vi "Get Variant Data From File.vi"(8 "error in (no error)":errorcluster, 10 "Variant Name":string, 11 "File refnum in":T1) -> (0 "error out":errorcluster, 2 "Variant Data Cluster":T2, 3 "File refnum out":T1)   [LabVIEW 2015]
uses:
  <vilib>/Utility/config.llb/Config Data RefNum.ctl
  Type defs/Variant Data Cluster.ctl
  <vilib>/Utility/config.llb/Read Key (String).vi
  <vilib>/Utility/config.llb/NI_LVConfig.lvlib
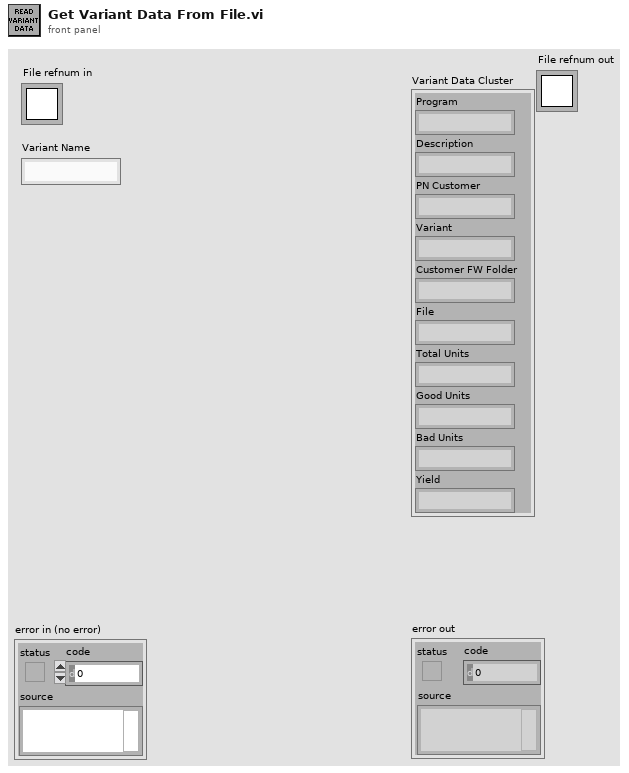
[diagram p1: front panel]
types:
  T1 = typedef "NI_LVConfig.lvlib/Config Data RefNum.ctl" = refnum<k1>
  T2 = typedef "Variant Data Cluster.ctl" = cluster{"Program":string, "Description":string, "PN Customer":string, "Variant":string, "Customer FW Folder":string, "File":string, "Total Units":string, "Good Units":string, "Bad Units":string, "Yield":string}
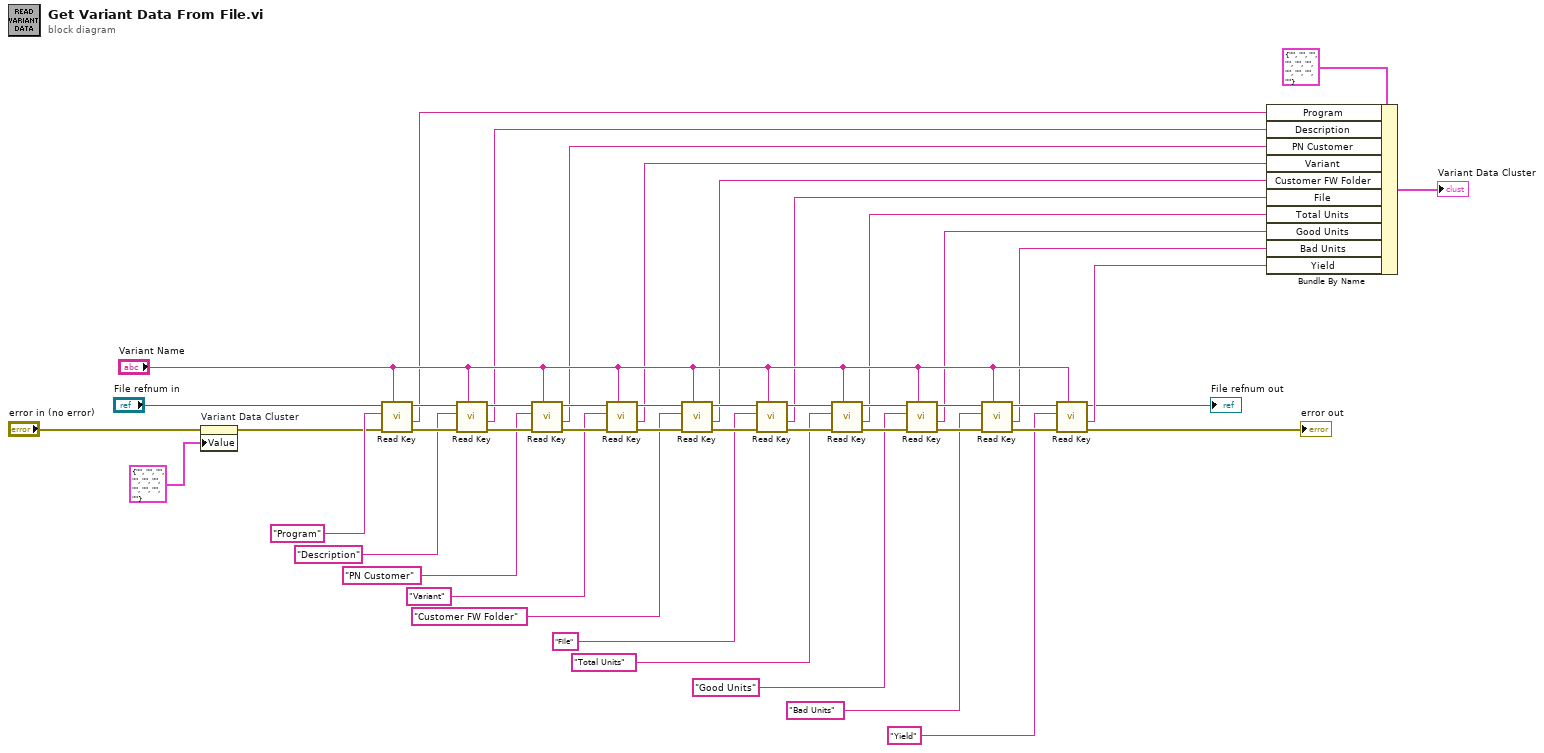
[diagram p0: block diagram]
diagram:
  n1 = property on="Variant Data Cluster" class="Clust (strict)"(error in="error in (no error)", "Value"=T2 {"Program"="", "Description"="", "PN Customer"="", "Variant"="", "Customer FW Folder"="", "File"="", "Total Units"="", "Good Units"="", "Bad Units"="", "Yield"=""} ("Variant Data Cluster")) -> (error out=w2:errorcluster)  [unwired: 1 in, 1 out]
  n2 = call-poly <vilib>:"Read Key.vi"("section"="Variant Name", "error in (no error)"=w2, "key"="Program", "refnum"="File refnum in") -> ("error out"=w43:errorcluster, "value"=w16:string, "refnum out"=w44:T1)  [unwired: 4 in, 1 out]
  n3 = call-poly <vilib>:"Read Key.vi"("section"="Variant Name", "error in (no error)"=w43, "key"="Description", "refnum"=w44) -> ("error out"=w42:errorcluster, "value"=w15:string, "refnum out"=w34:T1)  [unwired: 4 in, 1 out]
  n4 = call-poly <vilib>:"Read Key.vi"("section"="Variant Name", "error in (no error)"=w42, "key"="PN Customer", "refnum"=w34) -> ("error out"=w41:errorcluster, "value"=w14:string, "refnum out"=w33:T1)  [unwired: 4 in, 1 out]
  n5 = call-poly <vilib>:"Read Key.vi"("section"="Variant Name", "error in (no error)"=w41, "key"="Variant", "refnum"=w33) -> ("error out"=w40:errorcluster, "value"=w13:string, "refnum out"=w32:T1)  [unwired: 4 in, 1 out]
  n6 = call-poly <vilib>:"Read Key.vi"("section"="Variant Name", "error in (no error)"=w40, "key"="Customer FW Folder", "refnum"=w32) -> ("error out"=w39:errorcluster, "value"=w12:string, "refnum out"=w31:T1)  [unwired: 4 in, 1 out]
  n7 = call-poly <vilib>:"Read Key.vi"("section"="Variant Name", "error in (no error)"=w39, "key"="File", "refnum"=w31) -> ("error out"=w38:errorcluster, "value"=w11:string, "refnum out"=w30:T1)  [unwired: 4 in, 1 out]
  n8 = call-poly <vilib>:"Read Key.vi"("section"="Variant Name", "error in (no error)"=w38, "key"="Total Units", "refnum"=w30) -> ("error out"=w37:errorcluster, "value"=w10:string, "refnum out"=w29:T1)  [unwired: 4 in, 1 out]
  n9 = call-poly <vilib>:"Read Key.vi"("section"="Variant Name", "error in (no error)"=w37, "key"="Good Units", "refnum"=w29) -> ("error out"=w36:errorcluster, "value"=w9:string, "refnum out"=w28:T1)  [unwired: 4 in, 1 out]
  n10 = call-poly <vilib>:"Read Key.vi"("section"="Variant Name", "error in (no error)"=w36, "key"="Bad Units", "refnum"=w28) -> ("error out"=w35:errorcluster, "value"=w8:string, "refnum out"=w27:T1)  [unwired: 4 in, 1 out]
  n11 = call-poly <vilib>:"Read Key.vi"("section"="Variant Name", "error in (no error)"=w35, "key"="Yield", "refnum"=w27) -> ("error out"=→"error out":errorcluster, "value"=w7:string, "refnum out"=→"File refnum out":T1)  [unwired: 4 in, 1 out]
  n12 = Bundle By Name(cluster=T2 {"Program"="", "Description"="", "PN Customer"="", "Variant"="", "Customer FW Folder"="", "File"="", "Total Units"="", "Good Units"="", "Bad Units"="", "Yield"=""} ("Variant Data Cluster"), "Program"=w16, "Description"=w15, "PN Customer"=w14, "Variant"=w13, "Customer FW Folder"=w12, "File"=w11, "Total Units"=w10, "Good Units"=w9, "Bad Units"=w8, "Yield"=w7) -> (→"Variant Data Cluster":T2)
